vi "04-获取信号值.vi"   [LabVIEW 2015]
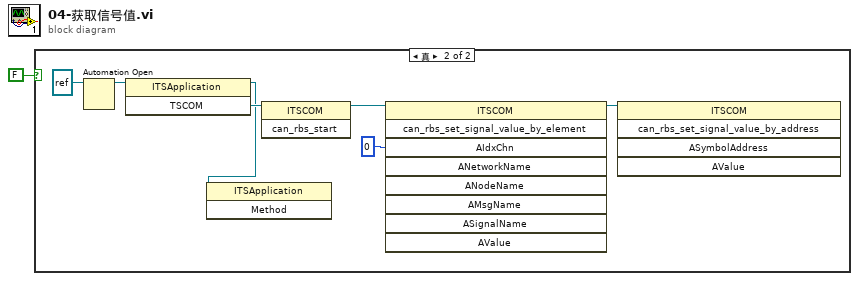
[diagram p0: block diagram]
diagram:
  n1 = case shown="真" FALSE {
    frame False {
    }
    frame True {
      n2 = Automation Open(Automation Refnum=refnum<k7> refnum ("comTSMaster.ITSApplication")) -> (Automation Refnum=w7:refnum<k7>)  [unwired: 3 in, 1 out]
      n3 = invoke on="调用节点" class="ITSApplication" method="TSCOM"(reference=w7) -> (reference out=w2:refnum<k7>, "TSCOM"=w6:refnum<k7>)  [unwired: 2 in, 1 out]
      n4 = invoke on="调用节点" class="ITSApplication" method=#-1(reference=w2) -> ()  [unwired: 2 in, 3 out]
      n5 = invoke on="调用节点" class="ITSCOM" method="can_rbs_start"(reference=w6) -> (reference out=w5:refnum<k7>)  [unwired: 2 in, 2 out]
      n6 = invoke on="调用节点" class="ITSCOM" method="can_rbs_set_signal_value_by_element"(reference=w5, "AIdxChn"=0) -> (reference out=w4:refnum<k7>)  [unwired: 7 in, 8 out]
      n7 = invoke on="调用节点" class="ITSCOM" method="can_rbs_set_signal_value_by_address"(reference=w4) -> ()  [unwired: 4 in, 5 out]
    }
  }
